vi "GetPathToModule.vi"(11 "module name":string="PythonNodeExamples.py") -> (3 "path to module":path)   [LabVIEW 2018]
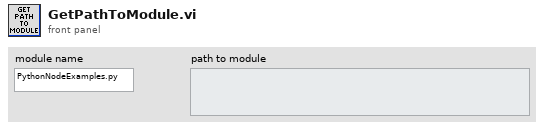
[diagram p1: front panel]
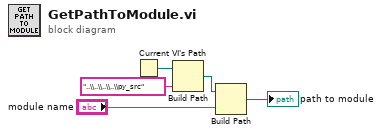
[diagram p0: block diagram]
diagram:
  n1 = Current VI's Path() -> (path=w4:path)
  n2 = Build Path(base path=w4, name or relative path="..\\..\\..\\..\\py_src") -> (appended path=w3:path)
  n3 = Build Path(base path=w3, name or relative path="module name") -> (appended path=→"path to module":path)
